vi "Free Memory Use.vi"(8 "error in":errorcluster, 10 "Cache Length":i32, 11 "MDPtr DVR":refnum<data-value>) -> (0 "error out":errorcluster)   [LabVIEW 2017, in "MDPtr.lvlib" / "MDPtrMgr.lvclass"]
uses:
  MDPtrMgr.lvclass
  MDPtr TypeDef/MDPtr DataFrame-Memory.ctl
  MDPtr TypeDef/MDPtr DataFrame-Common.ctl
  <vilib>/Utility/Data Type/Type Definitions/Data Type.ctl
  MDPtr.lvlib
  <vilib>/Utility/Data Type/NI_Data Type.lvlib
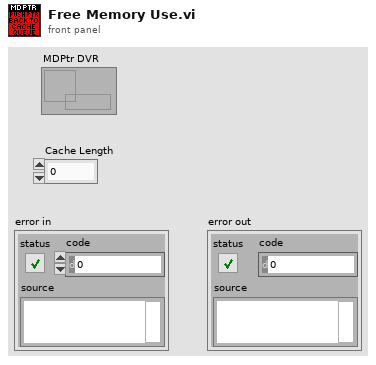
[diagram p1: front panel]
types:
  T1 = typedef "MDPtr.lvlib/MDPtr Queue.ctl" = refnum<queue>
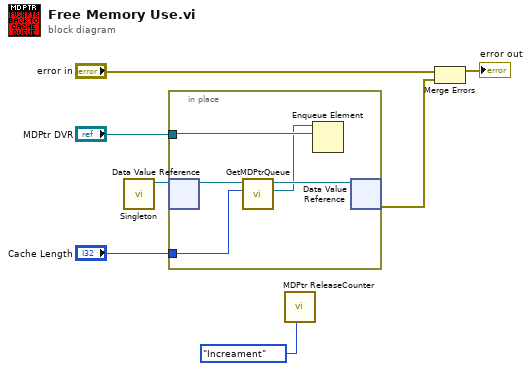
[diagram p0: block diagram]
diagram:
  n1 = call "Singleton.vi"() -> ("MDPtrMgrDVR"=w5:refnum<data-value>)  [unwired: 9 in, 2 out]
  n2 = in-place {
    in-place-border: "Cache Length" -> [w10]
    in-place-border: "MDPtr DVR" -> [w9]
    n3 = in-place-dvr #1(w5) -> (w12:refnum<class "MDPtrMgr.lvclass">)  [unwired: 1 out]
    n4 = call "GetMDPtrQueue.vi"("CacheSize"=w10, "MDPtrMgr in"=w12) -> ("MDPtrQueue"=w8:T1, "MDPtrMgr out"=w11:refnum<class "MDPtrMgr.lvclass">)  [unwired: 6 in, 2 out]
    n5 = Enqueue Element(queue=w8, element=w9) -> ()  [unwired: 2 in, 3 out]
    n6 = in-place-dvr #1(w11) -> (w1:errorcluster)  [unwired: 1 out]
  }
  n7 = call "MDPtr ReleaseCounter.vi"("Oper(Get)"=enum16{"GET", "Increament", "decreament"}."Increament") -> ()  [unwired: 9 in, 2 out]
  n8 = Merge Errors("error in", w1) -> (→"error out":errorcluster)
